vi "WhichValChanged.vi"() -> ()   [LabVIEW 2012]
panel:
  in  "Set00":bool
  in  "String":string
  out "Val Change Found":bool
  out "Val Change Event":bool
  in  "stop":bool=TRUE
  out "Col changed":i32
  out "Row Changed":i32
  out "Old table":string[][](table)=[["a", "e", "i", "m"], ["b", "f", "j", "n"], ["c", "g", "k", "o"], ["d", "h", "l", "p"]]
  in  "Table Control":string[][](table)=[["a", "e", "i", "m"], ["b", "f", "j", "n"], ["c", "g", "k", "o"], ["d", "h", "l", "p"]]
  # "Note: if change *adds* row/col, the displayed row/col changed will be new array size!"
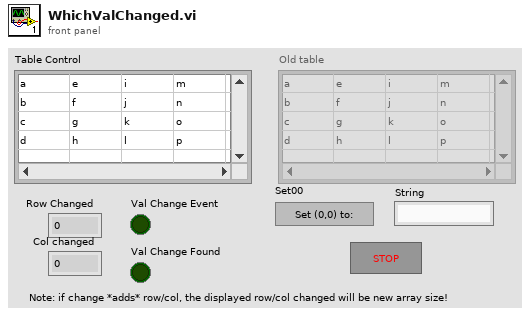
[diagram p1: front panel]
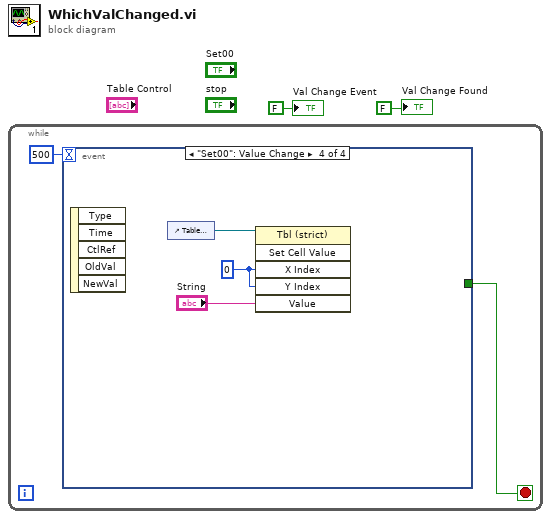
[diagram p0: block diagram]
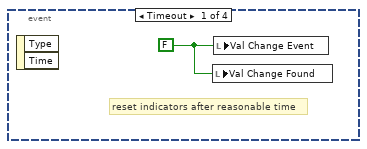
[diagram p2: hidden frame]
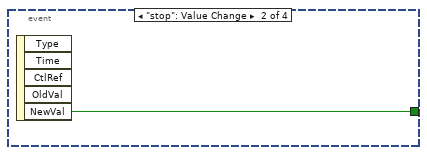
[diagram p3: hidden frame]
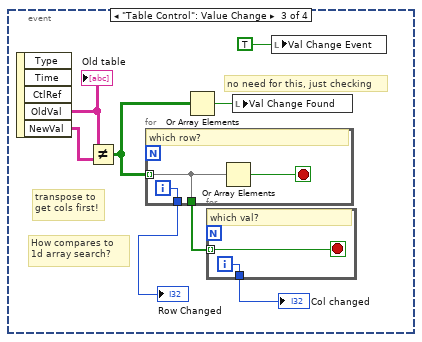
[diagram p4: hidden frame]
diagram:
  n1 = while {
    stop <- w4 stop-if-true
    n2 = event shown="[3] \"Set00\": Value Change" {
      selector: _ -> [_ _ _ _]
      dyn-events: _ -> [_ _ _ _]
      timeout: 500 -> [_ _ _ _]
      tunnel: [_ w6 _ _] -> w4
      event Timeout {
        w5 = FALSE
        # "reset indicators after reasonable time"
        n3 = event-data() -> ()  [unwired: 1 in, 2 out]
        n4 = local write "Val Change Found"(w5) -> ()
        n5 = local write "Val Change Event"(w5) -> ()
      }
      event "stop": Value Change {
        n6 = event-data() -> ("NewVal"=w6:bool)  [unwired: 1 in, 4 out]
      }
      event "Table Control": Value Change {
        # "no need for this, just checking"
        # "How compares to \n1d array search?"
        # "transpose to \nget cols first!"
        n7 = event-data() -> ("OldVal"=w13:string[][], "NewVal"=w12:string[][])  [unwired: 1 in, 3 out]
        "Old table" <- w13
        n8 = Not Equal?(x=w13, y=w12) -> (x != y?=w10:bool[][])
        n9 = for {
          tunnel: w10 -> [w18] mode=indexing
          tunnel: [w18] -> w9
          tunnel: [w17] -> w8
          i -> [w17]
          stop <- w19 stop-if-true
          # "which row?"
          n10 = Or Array Elements(Boolean array=w18) -> (logical OR=w19:bool)
        }
        "Row Changed" <- w8
        n11 = Or Array Elements(Boolean array=w10) -> (logical OR=w11:bool)
        n12 = for {
          tunnel: w9 -> [w16] mode=indexing
          tunnel: [w15] -> w7
          i -> [w15]
          stop <- w16 stop-if-true
          # "which val?"
        }
        "Col changed" <- w7
        n13 = local write "Val Change Found"(w11) -> ()
        n14 = local write "Val Change Event"(TRUE ("Val Change Event")) -> ()
      }
      event "Set00": Value Change {
        w20 = 0 ("X Index")
        n15 = event-data() -> ()  [unwired: 1 in, 5 out]
        n16 = control-ref of="Table Control"() -> (w22:refnum<vi>)
        n17 = invoke class="Tbl (strict)" method="Set Cell Value"(reference=w22, "X Index"=w20, "Y Index"=w20, "Value"="String") -> ()  [unwired: 2 in, 6 out]
      }
    }
  }
  "Val Change Found" <- FALSE
  "Val Change Event" <- FALSE ("Val Change Event")
